vi "Explore States Dialog.vi"(5 "Calling VI Ref":refnum<vi>, 8 "error in (no error)":errorcluster, 9 "StringConstant":refnum<vi>, 11 "JKI SM in":refnum<class "JKI SM.lvclass">) -> (0 "error out":errorcluster)   [LabVIEW 2020]
uses:
  JKI State Machine API/source/JKI SM/JKI SM.lvclass
  <userlib>/_OpenG.lib/error/error.llb/Filter Error Codes (Array)__ogtk.vi
  <vilib>/regexp/Match Regular Expression.xnode
  <userlib>/_OpenG.lib/comparison/comparison.llb/openg_comparison__ogtk.lvlib
  <userlib>/_OpenG.lib/comparison/comparison.llb/I32 Changed__ogtk.vi
  <userlib>/_OpenG.lib/comparison/comparison.llb/Boolean Changed__ogtk.vi
  <userlib>/_OpenG.lib/error/error.llb/openg_error.lvlib
  <userlib>/_OpenG.lib/string/string.llb/openg_string.lvlib
panel:
  in  "Listbox":i32(listbox)
  in  "OK":bool
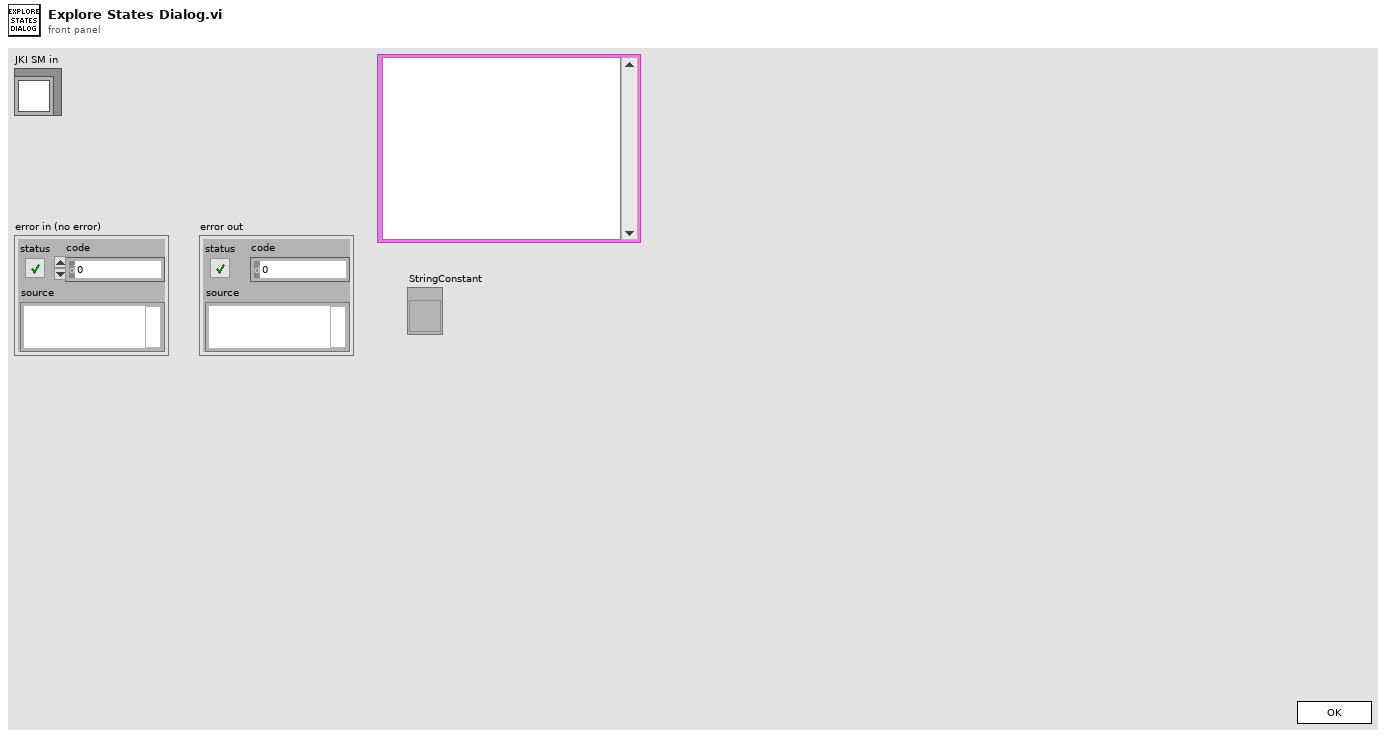
[diagram p1: front panel]
types:
  T1 = enum32{"Invalid", "Standard", "Closed", "Hidden", "Minimized", "Maximized"}
  T2 = enum32{"invalid app kind", "Development System", "Run Time System", "Student Edition", "Embedded LabVIEW", "Evaluation", "Custom"}
  T3 = enum32{"Invalid", "Default", "Floating", "Floating/Auto-Hide", "Modal"}
  T4 = cluster{"Core":cluster{"Current VI Reference":refnum<vi>, "Close Panel on Exit?":bool}, "Your Boolean data":bool, "Originating State":string, "JKI SM out":refnum<class "JKI SM.lvclass">, "States":string[], "StringConstant":refnum<vi>}
  T5 = cluster{"StringConstant":refnum<vi>, "Action":string, "Action":string}
  T6 = typedef "LVPoint32TypeDef.ctl" = cluster{"Horizontal":i32, "Vertical":i32}
  T7 = cluster{"Shift":bool, "Ctrl":bool, "Alt":bool, "Cmd":bool, "Opt":bool}
  T8 = cluster{"StringConstant":refnum<vi>, "Structure":string, "Frame Name":string, "State Call":string}[]
  T9 = cluster{"Current VI Reference":refnum<vi>, "Close Panel on Exit?":bool}
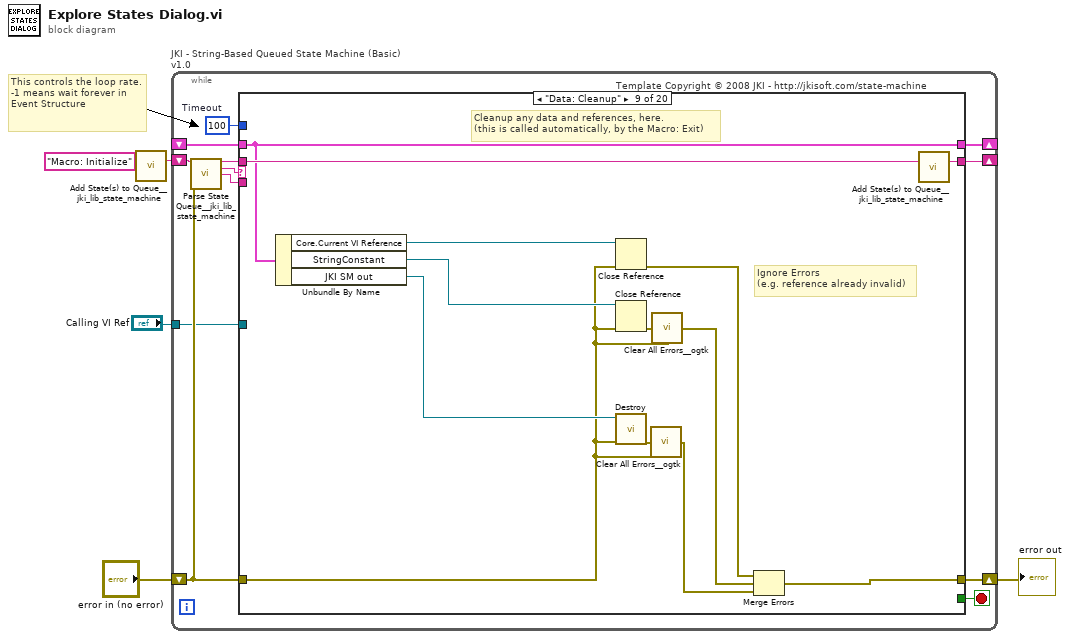
[diagram p0: block diagram]
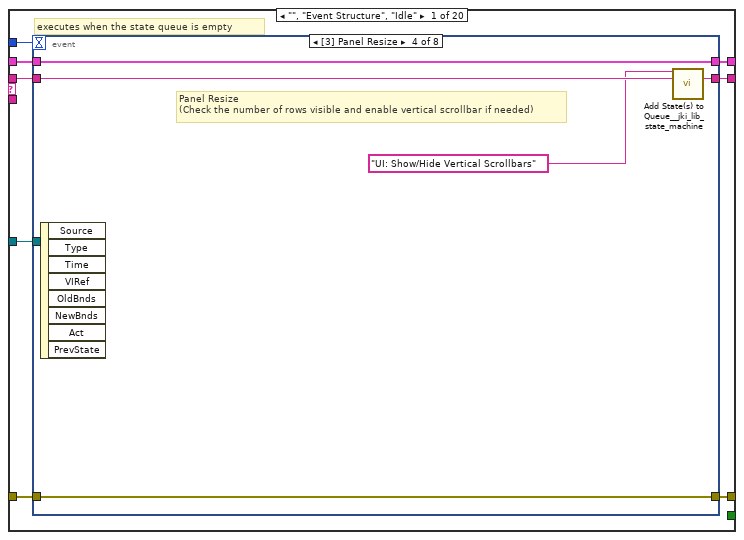
[diagram p2: hidden frame]
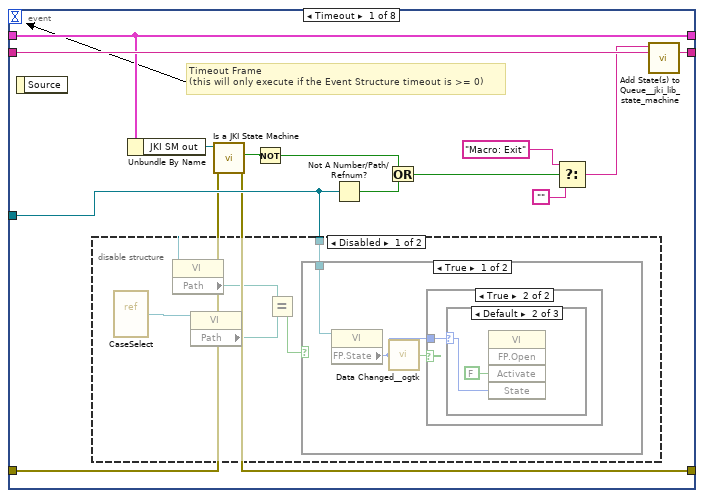
[diagram p3: hidden frame]
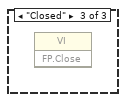
[diagram p6: hidden frame]
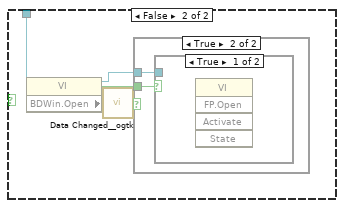
[diagram p7: hidden frame]
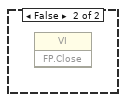
[diagram p9: hidden frame]
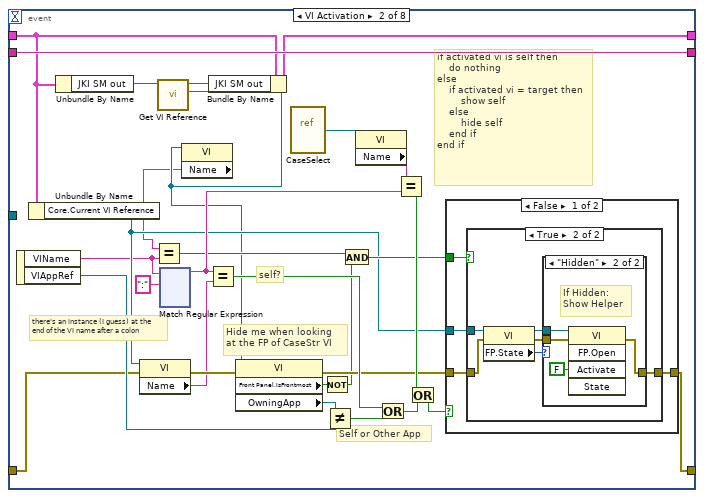
[diagram p11: hidden frame]
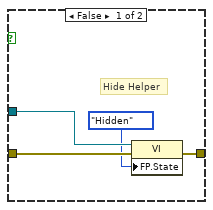
[diagram p12: hidden frame]
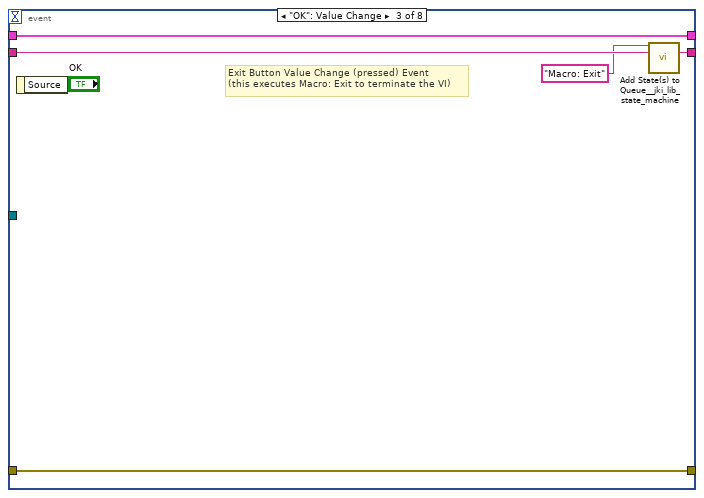
[diagram p15: hidden frame]
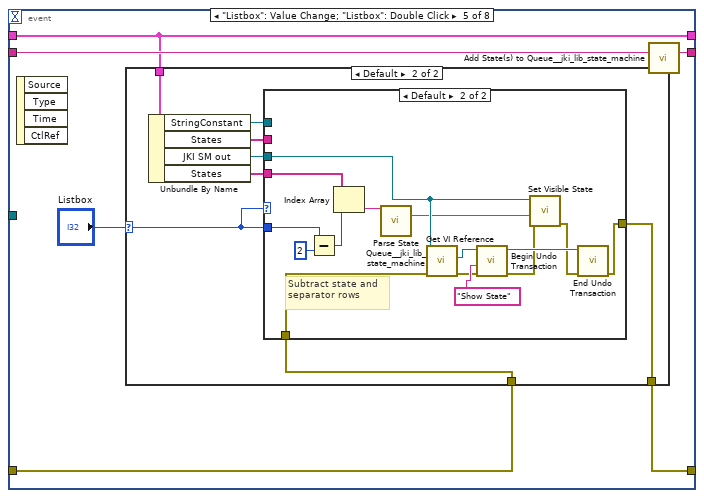
[diagram p16: hidden frame]
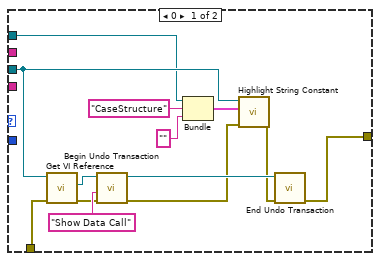
[diagram p18: hidden frame]
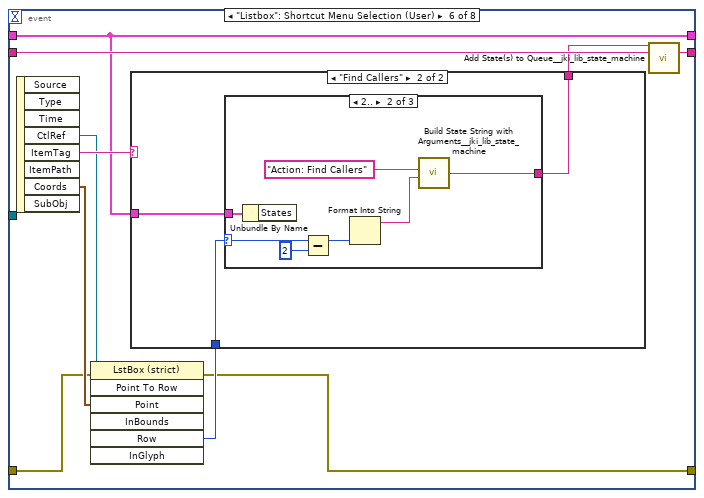
[diagram p19: hidden frame]
diagram:
  # "This controls the loop rate. -1 means wait forever in Event Structure"
  n1 = call <vilib>:"Add State(s) to Queue__jki_lib_state_machine.vi"("State(s) in (\"\")"="Macro: Initialize") -> ("States Out"=w5:string)  [unwired: 14 in]
  n2 = while "JKI - String-Based Queued State Machine (Basic) v1.0" {
    shift-right: [w10] -> _
    shift-left: _ -> [w9]
    shift-right: [w13] -> w3
    shift-left: "error in (no error)" -> [w7]
    shift-right: [w12] -> _
    shift-left: w5 -> [w14]
    tunnel: "Calling VI Ref" -> [w6]
    stop <- w11 stop-if-true
    w8 = 100  # Timeout
    # "Template Copyright © 2008 JKI - http://jkisoft.com/state-machine"
    n3 = call <vilib>:"Parse State Queue__jki_lib_state_machine.vi"("State Queue"=w14, "Error In (no error)"=w7) -> ("Remaining States"=w16:string, "Current State"=w17:string, "Arguments"=w15:string)  [unwired: 11 in]
    n4 = case shown="\"Data: Cleanup\"" w17 {
      selector: w17 -> [_ _ w380 _ _ _ _ _ _ _ _ _ _ _ _ _ _ _ _ _]
      tunnel: w16 -> [w25 w379 w384 w404 w415 w420 w424 w440 w453 w457 w469 w502 w527 w552 w563 w592 w597 w607 w611 w627]
      tunnel: w15 -> [_ _ _ _ _ _ _ _ _ _ _ _ _ w547 w557 _ _ _ _ w625]
      tunnel: w9 -> [w23 w376 w382 w396 w412 w418 w421 _ w450 w454 w461 w499 w521 w550 w559 w589 w595 w604 w608 w622]
      tunnel: [w22 w377 w386 w391 errorcluster {"status"=FALSE, "code"=0, "source"=""} ("error out") w417 w422 w431 w447 w455 w458 w496 w518 w548 w560 w590 w593 w605 w609 w617] -> w13
      tunnel: w7 -> [w21 w377 w385 w392 w410 w417 w422 w426 w442 w455 w459 w492 w519 w549 w561 w590 w593 w605 w609 w614]
      tunnel: [w24 w378 w383 w403 w414 w419 w423 w439 w452 w456 w468 w501 w526 w551 w562 w591 w596 w606 w610 w626] -> w12
      tunnel: [_ _ _ _ _ TRUE _ _ _ _ _ _ _ _ _ _ _ _ _ _] -> w11
      tunnel: [w20 w376 w382 w402 w412 w418 w421 w438 w450 w454 w461 w475 w521 w550 w559 w589 w595 w604 w608 w622] -> w10
      tunnel: w8 -> [w19 _ _ _ _ _ _ _ _ _ _ _ _ _ _ _ _ _ _ _]
      tunnel: w6 -> [w18 _ _ _ _ _ _ _ _ _ _ _ _ _ _ _ _ _ _ w616]
      frame "", "Event Structure", "Idle" {
        # "executes when the state queue is empty"
        n5 = event shown="[3] Panel Resize" {
          selector: _ -> [_ _ _ _ _ _ _ _]
          dyn-events: _ -> [_ _ _ _ _ _ _ _]
          timeout: w19 -> [_ _ _ _ _ _ _ _]
          tunnel: w25 -> [w39 w85 w221 w226 w232 w279 w302 w375]
          tunnel: [w38 w85 w220 w225 w231 w278 w301 w374] -> w24
          tunnel: w23 -> [w33 w59 w218 w223 w230 w270 w300 w372]
          tunnel: [w28 w60 w219 w224 w228 w271 w295 w373] -> w22
          tunnel: w21 -> [w29 w61 w219 w224 w229 w273 w296 w373]
          tunnel: [w33 w58 w218 w223 w230 w270 w300 w372] -> w20
          tunnel: w18 -> [w34 _ _ _ _ _ _ _]
          event Timeout {
            # "Timeout Frame\n(this will only execute if the Event Structure timeout is >= 0)"
            n6 = event-data() -> ()  [unwired: 1 in, 1 out]
            n7 = disable-structure shown="Disabled" {
              disable-tunnel: w34 -> [w40 _]
              frame Disabled {
                n8 = vi-ref "CaseSelect.vi"() -> (w42:refnum<vi>)
                n9 = property class="VI"(reference=w40) -> ("Path"=w41:path)  [unwired: 1 in, 2 out]
                n10 = property class="VI"(reference=w42) -> ("Path"=w44:path)  [unwired: 1 in, 2 out]
                n11 = Equal?(x=w41, y=w44) -> (x = y?=w43:bool)
                n12 = case shown="True" w43 {
                  tunnel: w40 -> [w45 w52]
                  frame True {
                    n13 = property class="VI"(reference=w45) -> ("FP.State"=w46:T1)  [unwired: 1 in, 2 out]
                    n14 = call-poly <userlib>:"Data Changed__ogtk.vi"("I32"=w46) -> ("Changed"=w47:bool)
                    n15 = case shown="True" w47 {
                      tunnel: w46 -> [_ w48]
                      frame False {
                      }
                      frame True {
                        n16 = case shown="Default" w48 {
                          selector: w48 -> [_ w49 _]
                          frame "Invalid" {
                          }
                          frame Default {
                            n17 = invoke class="VI" method="FP.Open"("Activate"=FALSE ("Activate?"), "State"=w49) -> ()  [unwired: 3 in, 5 out]
                          }
                          frame "Closed" {
                            n18 = invoke class="VI" method="FP.Close"() -> ()  [unwired: 3 in, 3 out]
                          }
                        }
                      }
                    }
                  }
                  frame False {
                    n19 = property class="VI"(reference=w52) -> (reference out=w51:refnum<vi>, "BDWin.Open"=w53:bool)  [unwired: 1 in, 1 out]
                    n20 = call-poly <userlib>:"Data Changed__ogtk.vi"("Boolean"=w53) -> ("Changed"=w54:bool)
                    n21 = case shown="True" w54 {
                      tunnel: w53 -> [_ w56]
                      tunnel: w51 -> [_ w55]
                      frame False {
                      }
                      frame True {
                        n22 = case shown="True" w56 {
                          tunnel: w55 -> [_ _]
                          frame True {
                            n23 = invoke class="VI" method="FP.Open"() -> ()  [unwired: 5 in, 5 out]
                          }
                          frame False {
                            n24 = invoke class="VI" method="FP.Close"() -> ()  [unwired: 3 in, 3 out]
                          }
                        }
                      }
                    }
                  }
                }
              }
              frame Enabled {
              }
            }
            n25 = Unbundle By Name(w33) -> ("JKI SM out"=w32:refnum<class "JKI SM.lvclass">)
            n26 = call "Is a JKI State Machine.vi"("error in (no error)"=w29, "JKI SM in"=w32) -> ("error out"=w28:errorcluster, "Is a JKI State Machine"=w31:bool)  [unwired: 7 in, 1 out]
            n27 = Not(x=w31) -> (.not. x?=w30:bool)
            n28 = Not A Number/Path/Refnum?(number/path/refnum=w34) -> (NaN/Path/Refnum?=w27:bool)
            n29 = Or(x=w30, y=w27) -> (x .or. y?=w26:bool)
            n30 = Select(t="Macro: Exit", s=w26, f="") -> (s? t:f=w35:string)
            n31 = call <vilib>:"Add State(s) to Queue__jki_lib_state_machine.vi"("State(s) in Front (\"\")"=w35, "State(s) in (\"\")"=w39) -> ("States Out"=w38:string)  [unwired: 13 in]
          }
          event VI Activation {
            # "Self or Other App"
            # "self?"
            # "Hide me when looking\nat the FP of CaseStr VI"
            # "there's an instance (I guess) at the\nend of the VI name after a colon"
            # "if activated vi is self then\n    do nothing\nelse\n    if activated vi = target then\n        show self\n    else\n        hide self\n    end if\nend if"
            n32 = event-data() -> ("VIName"=w63:string, "VIAppRef"=w62:refnum<vi>)  [unwired: 1 in]
            n33 = Unbundle By Name(w59) -> ("Core.Current VI Reference"=w70:refnum<vi>)
            n34 = Unbundle By Name(w59) -> ("JKI SM out"=w66:refnum<class "JKI SM.lvclass">)
            n35 = property class="VI"(reference=w70, error in=w61) -> (error out=w74:errorcluster, "Name"=w69:string)  [unwired: 1 out]
            n36 = call "Get VI Reference.vi"("JKI SM in"=w66) -> ("VI"=w65:refnum<vi>, "JKI SM out"=w57:refnum<class "JKI SM.lvclass">)  [unwired: 8 in, 1 out]
            n37 = xnode "Match Regular Expression"("input string"=w63, "regular expression"=":") -> ("before match"=w81:string)  [unwired: 3 in, 5 out]
            n38 = property class="VI"(reference=w65) -> ("Name"=w64:string)  [unwired: 1 in, 2 out]
            n39 = Equal?(x=w64, y=w63) -> (x = y?=w67:bool)
            n40 = Equal?(x=w81, y=w69) -> (x = y?=w78:bool)
            n41 = Bundle By Name(cluster=w59, "JKI SM out"=w57) -> (w58:T4)
            n42 = property class="VI"(reference=w65, error in=w74) -> (error out=w73:errorcluster, "Front Panel.IsFrontmost"=w71:bool, "OwningApp"=w76:refnum<vi>)  [unwired: 1 out]
            n43 = vi-ref "CaseSelect.vi"() -> (w79:refnum<vi>)
            n44 = Not(x=w71) -> (.not. x?=w72:bool)
            n45 = Not Equal?(x=w76, y=w62) -> (x != y?=w77:bool)
            n46 = And(x=w67, y=w72) -> (x .and. y?=w75:bool)
            n47 = property class="VI"(reference=w79) -> ("Name"=w80:string)  [unwired: 1 in, 2 out]
            n48 = Or(x=w78, y=w77) -> (x .or. y?=w83:bool)
            n49 = Equal?(x=w80, y=w81) -> (x = y?=w82:bool)
            n50 = Or(x=w82, y=w83) -> (x .or. y?=w84:bool)
            n51 = case shown="False" w84 {
              tunnel: w73 -> [w89 w105]
              tunnel: [w87 w105] -> w60
              tunnel: w70 -> [w88 _]
              tunnel: w75 -> [w86 _]
              frame False {
                n52 = case shown="True" w86 {
                  tunnel: w89 -> [w93 w98]
                  tunnel: w88 -> [w92 w99]
                  tunnel: [w91 w96] -> w87
                  frame False {
                    # "Hide Helper"
                    n53 = property class="VI"(reference=w92, error in=w93, "FP.State"=T1."Hidden" ("Front Panel Window:State")) -> (error out=w91:errorcluster)  [unwired: 1 out]
                  }
                  frame True {
                    n54 = property class="VI"(reference=w99, error in=w98) -> (reference out=w95:refnum<vi>, error out=w94:errorcluster, "FP.State"=w97:T1)
                    n55 = case shown="\"Hidden\"" w97 {
                      tunnel: [w100 w104] -> w96
                      tunnel: w95 -> [_ w103]
                      tunnel: w94 -> [w100 w102]
                      frame Default {
                      }
                      frame "Hidden" {
                        # "If Hidden:\nShow Helper"
                        n56 = invoke class="VI" method="FP.Open"(reference=w103, error in=w102, "Activate"=FALSE ("Activate?")) -> (error out=w104:errorcluster)  [unwired: 2 in, 4 out]
                      }
                    }
                  }
                }
              }
              frame True {
              }
            }
          }
          event "OK": Value Change {
            # "Exit Button Value Change (pressed) Event\n(this executes Macro: Exit to terminate the VI)"
            n57 = event-data() -> ()  [unwired: 1 in, 1 out]
            n58 = call <vilib>:"Add State(s) to Queue__jki_lib_state_machine.vi"("State(s) in Front (\"\")"="Macro: Exit", "State(s) in (\"\")"=w221) -> ("States Out"=w220:string)  [unwired: 13 in]
          }
          event Panel Resize {
            # "Panel Resize\n(Check the number of rows visible and enable vertical scrollbar if needed)"
            n59 = event-data() -> ()  [unwired: 1 in, 8 out]
            n60 = call <vilib>:"Add State(s) to Queue__jki_lib_state_machine.vi"("State(s) in Front (\"\")"="UI: Show/Hide Vertical Scrollbars" ("State(s) in Front (\"\")"), "State(s) in (\"\")"=w226) -> ("States Out"=w225:string)  [unwired: 13 in]
          }
          event "Listbox": Value Change; "Listbox": Double Click {
            n61 = event-data() -> ()  [unwired: 1 in, 4 out]
            n62 = case shown="Default" "Listbox" {
              selector: "Listbox" -> [_ w235]
              tunnel: w230 -> [_ w241]
              tunnel: w229 -> [w233 w238]
              tunnel: [w233 w237] -> w228
              frame -1 {
              }
              frame Default {
                n63 = Unbundle By Name(w241) -> ("StringConstant"=w234:refnum<vi>, "States"=w236:string[], "JKI SM out"=w239:refnum<class "JKI SM.lvclass">, "States"=w240:string[])
                n64 = case shown="Default" w235 {
                  tunnel: w240 -> [_ w269]
                  tunnel: w239 -> [w253 w262]
                  tunnel: w238 -> [w254 w258]
                  tunnel: w235 -> [_ w267]
                  tunnel: [w252 w259] -> w237
                  tunnel: w236 -> [_ _]
                  tunnel: w234 -> [w251 _]
                  frame 0 {
                    n65 = call "Get VI Reference.vi"("error in (no error)"=w254, "JKI SM in"=w253) -> ("error out"=w249:errorcluster, "VI"=w248:refnum<vi>)  [unwired: 7 in, 1 out]
                    n66 = call "Begin Undo Transaction.vi"("error in (no error)"=w249, "Action"="Show Data Call", "VI in"=w248) -> ("error out"=w245:errorcluster, "VI out"=w247:refnum<vi>)  [unwired: 7 in]
                    n67 = Bundle("StringConstant"=w251, "Action"="CaseStructure", "Action"="") -> (w244:T5)  [unwired: 1 in]
                    n68 = call "Highlight String Constant.vi"("error in (no error)"=w245, "Cluster"=w244, "JKI SM in"=w253) -> ("error out"=w246:errorcluster)  [unwired: 7 in, 1 out]
                    n69 = call "End Undo Transaction.vi"("error in (no error)"=w246, "VI in"=w247) -> ("error out"=w252:errorcluster)  [unwired: 8 in, 1 out]
                  }
                  frame Default {
                    # "Subtract state and separator rows"
                    n70 = Subtract(x=w267, y=2) -> (x-y=w266:i32)
                    n71 = Index Array(array=w269, index=w266) -> (element=w256:string)
                    n72 = call <vilib>:"Parse State Queue__jki_lib_state_machine.vi"("State Queue"=w256) -> ("Current State"=w255:string)  [unwired: 12 in, 2 out]
                    n73 = call "Get VI Reference.vi"("error in (no error)"=w258, "JKI SM in"=w262) -> ("error out"=w264:errorcluster, "VI"=w263:refnum<vi>)  [unwired: 7 in, 1 out]
                    n74 = call "Begin Undo Transaction.vi"("error in (no error)"=w264, "Action"="Show State", "VI in"=w263) -> ("error out"=w257:errorcluster, "VI out"=w261:refnum<vi>)  [unwired: 7 in]
                    n75 = call "Set Visible State.vi"("error in (no error)"=w257, "State Name"=w255, "JKI SM in"=w262) -> ("error out"=w260:errorcluster)  [unwired: 7 in, 1 out]
                    n76 = call "End Undo Transaction.vi"("error in (no error)"=w260, "VI in"=w261) -> ("error out"=w259:errorcluster)  [unwired: 8 in, 1 out]
                  }
                }
              }
            }
            n77 = call <vilib>:"Add State(s) to Queue__jki_lib_state_machine.vi"("State(s) in (\"\")"=w232) -> ("States Out"=w231:string)  [unwired: 14 in]
          }
          event "Listbox": Shortcut Menu Selection (User) {
            n78 = event-data() -> ("CtlRef"=w276:refnum<vi>, "ItemTag"=w277:string, "Coords"=w275:T6)  [unwired: 1 in, 5 out]
            n79 = invoke class="LstBox (strict)" method="Point To Row"(reference=w276, error in=w273, "Point"=w275) -> (error out=w271:errorcluster, "Row"=w274:i32)  [unwired: 4 in, 5 out]
            n80 = case shown="\"Find Callers\"" w277 {
              tunnel: w274 -> [_ w282]
              tunnel: [_ w281] -> w272
              tunnel: w270 -> [_ w280]
              frame Default {
              }
              frame "Find Callers" {
                n81 = case shown="2.." w282 {
                  selector: w282 -> [_ w286 _]
                  tunnel: [_ w287 w290] -> w281
                  tunnel: w280 -> [_ w283 _]
                  frame -1, Default {
                  }
                  frame 2.. {
                    n82 = Unbundle By Name(w283) -> ()  [unwired: 1 out]
                    n83 = Subtract(x=w286, y=2) -> (x-y=w285:i32)
                    n84 = Format Into String(w285) -> (resulting string=w288:string)  [unwired: 3 in, 1 out]
                    n85 = call <vilib>:"Build State String with Arguments__jki_lib_state_machine.vi"("Arguments (\"\")"=w288, "State"="Action: Find Callers") -> ("State with Arguments"=w287:string)  [unwired: 4 in]
                  }
                  frame 0 {
                    n86 = disable-structure shown="Disabled" {
                      disable-tunnel: [w291 _] -> w290
                      frame Disabled {
                        n87 = call <vilib>:"Build State String with Arguments__jki_lib_state_machine.vi"("State"="Action: Delete State") -> ("State with Arguments"=w291:string)  [unwired: 5 in]
                      }
                      frame Enabled {
                      }
                    }
                  }
                }
              }
            }
            n88 = call <vilib>:"Add State(s) to Queue__jki_lib_state_machine.vi"("State(s) in Front (\"\")"=w272, "State(s) in (\"\")"=w279) -> ("States Out"=w278:string)  [unwired: 13 in]
          }
          event Key Down? {
            n89 = event-data() -> ("Char"=w299:i16, "ScanCode"=w294:i16, "PlatMods"=w298:T7)  [unwired: 1 in, 7 out]
            n90 = case shown="Default" w294 {
              tunnel: w300 -> [_ w320]
              tunnel: w299 -> [_ w318]
              tunnel: w298 -> [_ w315]
              tunnel: [_ w313] -> w297
              tunnel: w296 -> [w304 w311]
              tunnel: [w304 w310] -> w295
              tunnel: [w303 _] -> w293
              frame 83 {
                n91 = local read "Listbox"() -> (w305:i32)
                n92 = case shown="Default" w305 {
                  selector: w305 -> [_ w306]
                  tunnel: [_ w307] -> w303
                  frame -1 {
                  }
                  frame Default {
                    n93 = Format Into String(w306) -> (resulting string=w308:string)  [unwired: 3 in, 1 out]
                    n94 = call <vilib>:"Build State String with Arguments__jki_lib_state_machine.vi"("Arguments (\"\")"=w308, "State"="Action: Delete State Call") -> ("State with Arguments"=w307:string)  [unwired: 4 in]
                  }
                }
              }
              frame Default {
                n95 = Unbundle By Name(w320) -> ("JKI SM out"=w312:refnum<class "JKI SM.lvclass">, "States"=w319:string[])
                n96 = Build Array(w318) -> (w317:i16[])
                n97 = Unbundle By Name(w315) -> ("Ctrl"=w314:bool)
                n98 = Byte Array To String(unsigned byte array=w317) -> (string=w316:string)
                n99 = case shown="True" w314 {
                  tunnel: w319 -> [_ w329]
                  tunnel: w316 -> [_ w328]
                  tunnel: w315 -> [_ w327]
                  tunnel: [_ w326] -> w313
                  tunnel: w312 -> [_ w324]
                  tunnel: [w321 w323] -> w310
                  tunnel: w311 -> [w321 w322]
                  frame False {
                  }
                  frame True {
                    n100 = To Upper Case(1:w328) -> (0:w325:string)
                    n101 = case shown="\"F\"" w325 {
                      tunnel: w329 -> [_ w344 w353 _]
                      tunnel: w327 -> [_ w339 _ w362]
                      tunnel: [_ TRUE TRUE TRUE] -> w326
                      tunnel: w324 -> [_ _ w347 w359]
                      tunnel: [w330 w337 w345 w356] -> w323
                      tunnel: w322 -> [w330 w337 w346 w360]
                      frame Default {
                      }
                      frame "G" {
                        w332 = 2 ("y")
                        n102 = local read "Listbox"() -> (w334:i32)
                        n103 = Unbundle By Name(w339) -> ("Shift"=w340:bool)
                        n104 = Array Size(array=w344) -> (size(s)=w331:i32)
                        n105 = Subtract(x=w334, y=w332) -> (x-y=w333:i32)
                        n106 = Decrement(x=w333) -> (x-1=w342:i32)
                        n107 = Increment(x=w333) -> (x+1=w343:i32)
                        n108 = Select(t=w342, s=w340, f=w343) -> (s? t:f=w341:i32)
                        n109 = Quotient & Remainder(x=w341, y=w331) -> (x-y*floor(x/y)=w336:i32)  [unwired: 1 out]
                        n110 = Add(x=w336, y=w332) -> (x+y=w335:i32)
                        n111 = property on="Listbox" class="LstBox (strict)"("Val(Sgnl)"=w335) -> ()  [unwired: 2 in, 2 out]
                      }
                      frame "F" {
                        n112 = local read "Listbox"() -> (w354:i32)
                        n113 = Index Array(array=w353, index=w354) -> (element=w352:string)
                        n114 = control-ref of="This VI"() -> (w348:refnum<vi>)
                        n115 = call "Find All Callers of State.vi"("error in (no error)"=w346, "State Name"=w352, "JKI SM in"=w347) -> ("error out"=w349:errorcluster, "Callers"=w350:T8, "JKI SM out"=w351:refnum<class "JKI SM.lvclass">)  [unwired: 6 in]
                        n116 = call "Open Search Results Dialog.vi"("VI Refnum"=w348, "error in (no error)"=w349, "Callers"=w350, "State"=w352, "JKI SM in"=w351) -> ("error out"=w345:errorcluster)  [unwired: 6 in]
                      }
                      frame "Z" {
                        # "Override Ctrl+Z and Ctrl+Shift+Z\n(Handle them here and target the user's VI)"
                        n117 = call "Get VI Reference.vi"("error in (no error)"=w360, "JKI SM in"=w359) -> ("error out"=w357:errorcluster, "VI"=w358:refnum<vi>)  [unwired: 7 in, 1 out]
                        n118 = Unbundle By Name(w362) -> ("Shift"=w361:bool)
                        n119 = case shown="False" w361 {
                          tunnel: w358 -> [w366 w369]
                          tunnel: w357 -> [w364 w368]
                          tunnel: [w365 w367] -> w356
                          frame False {
                            n120 = invoke class="VI" method="Transaction.Undo"(reference=w366, error in=w364) -> (error out=w365:errorcluster)  [unwired: 1 in, 2 out]
                          }
                          frame True {
                            n121 = invoke class="VI" method="Transaction.Redo"(reference=w369, error in=w368) -> (error out=w367:errorcluster)  [unwired: 1 in, 2 out]
                          }
                        }
                      }
                    }
                  }
                }
              }
            }
            n122 = event-data("Discard?"=w297) -> ()  [unwired: 1 in, 1 out]
            n123 = call <vilib>:"Add State(s) to Queue__jki_lib_state_machine.vi"("State(s) in Front (\"\")"=w293, "State(s) in (\"\")"=w302) -> ("States Out"=w301:string)  [unwired: 13 in]
          }
          event Panel Close? {
            # "Discard the event because we'll close the front panel ourselves in Macro: Exit"
            # "Close Panel button (pressed) Event\n(this executes Macro: Exit to terminate the VI)"
            n124 = event-data() -> ()  [unwired: 1 in, 1 out]
            n125 = event-data("Discard?"=TRUE) -> ()  [unwired: 1 in, 1 out]
            n126 = call <vilib>:"Add State(s) to Queue__jki_lib_state_machine.vi"("State(s) in Front (\"\")"="Macro: Exit", "State(s) in (\"\")"=w375) -> ("States Out"=w374:string)  [unwired: 13 in]
          }
        }
      }
      frame "---------- Core ----------" {
        # "Do not put any code in this frame.\n(it is a separator no-op)"
        n127 = call <vilib>:"Add State(s) to Queue__jki_lib_state_machine.vi"("State(s) in (\"\")"=w379) -> ("States Out"=w378:string)  [unwired: 14 in]
      }
      frame Default {
        w389 = 42 items=["No error", "Argument error", "Memory is full", "Out of zone", "End of file", "File already open", "Generic file I/O error", "File not found", "File permission error", "Disk is full", "Duplicate path", "Too many files open", "System feature not enabled", "Resource file not found", "Cannot add resource", "Resource not found", "Image not found", "Image memory error", "Pen does not exist", "Config type invalid", "Config token not found", "Config parse error", "Config memory error", "Bad external code format", "Bad external code offset", "External code not present", "Null window", "Destroy window error", "Null menu", "Print aborted", "Bad print record", "Print driver error", "Windows error during printing", "Memory error during printing", "Print dialog error", "Generic print error", "Invalid device refnum", "Device not found", "Device parameter error", "Device unit error", "Cannot open device", "Device call aborted", "Generic error", "Cancelled by user", "Object ID too low", "Object ID too high", "Object not in heap", "Unknown heap", "Unknown object (invalid DefProc)", "Unknown object (DefProc not in table)", "Message out of range", "Invalid (null) method", "Unknown message", "Manager call not supported", "Bad address", "Network operation in progress", "Network operation timed out", "Connection is busy", "Network attribute not supported", "Network error", "Address in use", "System out of memory", "Connection aborted", "Connection refused", "Not connected", "Already connected", "Connection closed", "Initialization error (interapplication manager)", "Bad occurrence", "Wait on unbound occurrence handler", "Occurrence queue overflow", "Datalog type conflict", "Unused", "Unrecognized type (interapplication manager)", "Memory corrupt", "Failed to make temporary DLL", "Old CIN version", "Drag socket not found", "Failed to load drop-object", "Failed to register OLE object", "Failed to release OLE object", "Format specifier type mismatch", "Unknown format specifier", "Too few format specifiers", "Too many format specifiers", "Scan failed", "Newer CIN version", "Error converting to variant", "Runtime menu error", "Password tampered", "Variant attribute not found", "Incompatible variant data type", "Event data is not available", "Event Store is not present", "Occurrence is not found", "Event Queue is not created", "Event info is not available", "Refnum passed is NULL", "Error retrieving Class GUID", "Error retrieving CoClass GUID", "Error retrieving TypeLib GUID.", "Bad built application magic bytes.", "Specific driver is different from the specific driver associated with the Logical Name.", "There is no session opened to the class driver.", "Max Error", "MAX - Error with config objects", "MAX - Error loading configuration", "MAX - Group not supported"]
        # "Current State"
        # "Do not delete, rename, or modify this frame.\n(this is used to capture unhandled states and typos)"
        # "Handle mistyped state name (developer tool)"
        n128 = Format Into String(format string="Software Exception: Unhandled State \"%s\"." ("message"), error in=w385, w380) -> (resulting string=w388:string, error out=w387:errorcluster)  [unwired: 1 in]
        n129 = call <vilib>:"Error Cluster From Error Code.vi"("show call chain? (False)"=TRUE, "error in (no error)"=w387, "error message (\"\")"=w388, "error code (0)"=w389) -> ("error out"=w386:errorcluster)  [unwired: 5 in]
        n130 = call <vilib>:"Add State(s) to Queue__jki_lib_state_machine.vi"("State(s) in (\"\")"=w384) -> ("States Out"=w383:string)  [unwired: 14 in]
      }
      frame "Initialize Core Data" {
        # "Do not delete, rename, or modify this frame.\n(this is used to determine panel behavior on exit)"
        # "originally closed?"
        # "exe?"
        # "If panel starts closed or is an EXE, then close it when we exit"
        n131 = property class="VI"() -> ("Clone Name"=w394:string)  [unwired: 2 in, 2 out]
        n132 = Open VI Reference(vi path=w394, error in (no error)=w392) -> (vi reference=w393:refnum<vi>, error out=w391:errorcluster)  [unwired: 4 in]
        n133 = property class="VI"() -> ("Front Panel.Open"=w401:bool)  [unwired: 2 in, 2 out]
        n134 = property class="App"() -> ("App.Kind"=w400:T2)  [unwired: 2 in, 2 out]
        n135 = Not(x=w401) -> (.not. x?=w398:bool)
        n136 = Equal?(x=w400, y=T2."Run Time System" ("Application:Kind")) -> (x = y?=w397:bool)
        n137 = Or(x=w398, y=w397) -> (x .or. y?=w395:bool)
        n138 = Bundle By Name(cluster=w396, "Core.Current VI Reference"=w393, "Core.Close Panel on Exit?"=w395) -> (w402:T4)
        n139 = call <vilib>:"Add State(s) to Queue__jki_lib_state_machine.vi"("State(s) in (\"\")"=w404) -> ("States Out"=w403:string)  [unwired: 14 in]
      }
      frame "Error Handler" {
        w411 = i32[] [1026]  # JKI SM VI Invalid Ref
        # "Unhandled Error -- Display it"
        # "Handle any errors here.\nYou can also output any states to clean-up after errors occur"
        # "Clear error"
        n140 = call-poly <userlib>:"Filter Error Codes__ogtk.vi"("Error In"=w410, "Error Codes to Filter"=w411) -> ("Error Out"=w409:errorcluster, "Error Filtered?"=w408:bool)  [unwired: 7 in, 1 out]
        n141 = call <vilib>:"General Error Handler.vi"("error in (no error)"=w409) -> ()  [unwired: 10 in, 5 out]
        n142 = Select(t="Macro: Exit", s=w408, f="") -> (s? t:f=w405:string)
        n143 = call <vilib>:"Add State(s) to Queue__jki_lib_state_machine.vi"("State(s) in Front (\"\")"=w405, "State(s) in (\"\")"=w415) -> ("States Out"=w414:string)  [unwired: 13 in]
      }
      frame "Exit" {
        # "Do not put any code in this frame.\n(No errors that occur here will be handled.)"
        n144 = call <vilib>:"Add State(s) to Queue__jki_lib_state_machine.vi"("State(s) in (\"\")"=w420) -> ("States Out"=w419:string)  [unwired: 14 in]
      }
      frame "---------- Data ----------" {
        # "Do not put any code in this frame.\n(It is a separator no-op. You can make a copy of this frame to create a new Data frame)"
        n145 = call <vilib>:"Add State(s) to Queue__jki_lib_state_machine.vi"("State(s) in (\"\")"=w424) -> ("States Out"=w423:string)  [unwired: 14 in]
      }
      frame "Data: Initialize" {
        w434 = string[] []  # States
        w435 = T9 {"Current VI Reference"=refnum, "Close Panel on Exit?"=FALSE}  # Core
        w437 = TRUE  # Your Boolean data
        w436 = ""  # Originating State
        # "do not delete - used by framework"
        # "Expand Bundle to add new data elements to shift register data."
        # "Add new data here."
        # "Data names and types of shift register data are defined by this bundle."
        # "Initialize the shift-register data, here.\n(data names are defined by what you wire into the bundle function)"
        n146 = call "Create (From State String Constant).vi"("error in (no error)"=w426, "State String Constant"="StringConstant") -> ("error out"=w425:errorcluster, "JKI SM out"=w427:refnum<class "JKI SM.lvclass">)  [unwired: 6 in, 2 out]
        n147 = property class="StrCnst"(reference="StringConstant", error in=w425) -> (error out=w432:errorcluster, "Text.Text"=w430:string)  [unwired: 1 out]
        n148 = call <userlib>:"Multi-line String to Array__ogtk.vi"("string"=w430) -> ("lines"=w429:string[])
        n149 = Variant To Data(error in=w432, type=w434, Variant=w429) -> (data=w433:string[], error out=w431:errorcluster)
        n150 = Bundle("Core"=w435, "Your Boolean data"=w437, "Originating State"=w436, "JKI SM out"=w427, "States"=w433, "StringConstant"="StringConstant") -> (w438:T4)  [unwired: 1 in]
        n151 = call <vilib>:"Add State(s) to Queue__jki_lib_state_machine.vi"("State(s) in (\"\")"=w440) -> ("States Out"=w439:string)  [unwired: 14 in]
      }
      frame "Data: Cleanup" {
        # "Ignore Errors\n(e.g. reference already invalid)"
        # "Cleanup any data and references, here.\n(this is called automatically, by the Macro: Exit)"
        n152 = Unbundle By Name(w450) -> ("Core.Current VI Reference"=w451:refnum<vi>, "StringConstant"=w449:refnum<vi>, "JKI SM out"=w443:refnum<class "JKI SM.lvclass">)
        n153 = Close Reference(reference=w451, error in (no error)=w442) -> (error out=w448:errorcluster)
        n154 = Close Reference(reference=w449, error in (no error)=w442) -> (error out=w446:errorcluster)
        n155 = call "Destroy.vi"("error in (no error)"=w442, "JKI SM in"=w443) -> ("error out"=w444:errorcluster)  [unwired: 9 in]
        n156 = call <userlib>:"Clear All Errors__ogtk.vi"("Upsteam Error (optional)"=w442, "Error In"=w444) -> ("Error Out"=w441:errorcluster)  [unwired: 2 in]
        n157 = call <userlib>:"Clear All Errors__ogtk.vi"("Upsteam Error (optional)"=w442, "Error In"=w446) -> ("Error Out"=w445:errorcluster)  [unwired: 2 in]
        n158 = Merge Errors(w448, w445, w441) -> (w447:errorcluster)
        n159 = call <vilib>:"Add State(s) to Queue__jki_lib_state_machine.vi"("State(s) in (\"\")"=w453) -> ("States Out"=w452:string)  [unwired: 14 in]
      }
      frame "---------- UI ----------" {
        # "Do not put any code in this frame.\n(It is a separator no-op. You can make a copy of this frame to create a new UI frame)"
        n160 = call <vilib>:"Add State(s) to Queue__jki_lib_state_machine.vi"("State(s) in (\"\")"=w457) -> ("States Out"=w456:string)  [unwired: 14 in]
      }
      frame "UI: Show/Hide Vertical Scrollbars" {
        # "Add +1 for the Parent Frame and another +1 for the horizontal divider"
        n161 = Unbundle By Name(w461) -> ("States"=w464:string[])
        n162 = Array Size(array=w464) -> (size(s)=w467:i32)
        n163 = property on="Listbox" class="LstBox (strict)"(error in=w459) -> (error out=w460:errorcluster, "Number of Rows"=w466:u32)  [unwired: 1 in, 1 out]
        n164 = Increment(x=w467) -> (x+1=w463:i32)
        n165 = Increment(x=w463) -> (x+1=w462:i32)
        n166 = Greater Or Equal?(x=w462, y=w466) -> (x >= y?=w465:bool)
        n167 = property on="Listbox" class="LstBox (strict)"(error in=w460, "Scrollbar Visible"=w465) -> (error out=w458:errorcluster)  [unwired: 1 in, 1 out]
        n168 = call <vilib>:"Add State(s) to Queue__jki_lib_state_machine.vi"("State(s) in (\"\")"=w469) -> ("States Out"=w468:string)  [unwired: 14 in]
      }
      frame "UI: Initialize" {
        # "Initialize the User Interface, here.\n(this is called automatically, by the Macro: Init)"
        n169 = Unbundle By Name(w499) -> ("Core.Current VI Reference"=w500:refnum<vi>, "States"=w471:string[], "JKI SM out"=w497:refnum<class "JKI SM.lvclass">, "StringConstant"=w498:refnum<vi>)
        n170 = property class="StrCnst"(reference=w498, error in=w492) -> (error out=w491:errorcluster, "Label.Text"=w488:string)  [unwired: 1 out]
        n171 = Empty String/Path?(string/path=w488) -> (empty?=w495:bool)
        n172 = call "Get State String Info.vi"("error in (no error)"=w491, "GObj Refnum in"=w498, "JKI SM in"=w497) -> ("error out"=w496:errorcluster, "Frame Name"=w490:string, "Structure"=w482:string)  [unwired: 5 in, 1 out]
        n173 = Not(x=w495) -> (.not. x?=w493:bool)
        n174 = Not Equal?(x=w490, y=w488) -> (x != y?=w494:bool)
        n175 = Equal?(x="EventStructure", y=w482) -> (x = y?=w483:bool)
        n176 = And(x=w494, y=w493) -> (x .and. y?=w489:bool)
        n177 = Build Array(w488) -> (w487:string[])
        n178 = Build Array(w482) -> (w481:string[])
        n179 = Select(t=w487, s=w489, f=string[] []) -> (s? t:f=w486:string[])
        n180 = Select(t=w481, s=w483, f=string[] []) -> (s? t:f=w479:string[])
        n181 = Build Array (concatenate)(w479, w490, w486) -> (w478:string[])
        n182 = call <userlib>:"1D Array to String__ogtk.vi"("delimiter (Tab)"=": ", "Array of Strings"=w478) -> ("delimited string"=w474:string)  [unwired: 9 in]
        n183 = Format Into String(format string="Back to %s", w474) -> (resulting string=w472:string)  [unwired: 2 in, 1 out]
        n184 = disable-structure shown="Enabled" {
          disable-tunnel: w471 -> [w504 w513]
          disable-tunnel: w472 -> [w503 _]
          frame Enabled {
            n185 = Build Array (concatenate)(w503, "" ("format string"), w504) -> (w510:string[])
            n186 = property on="Listbox" class="LstBox (strict)"("Item Names"=w510, "Value"=-1 ("Listbox")) -> (error out=w509:errorcluster, "Item Symbols"=w508:i32[])  [unwired: 2 in, 1 out]
            n187 = Replace Array Subset(array=w508, new element=-1 ("new element/subarray"), index=1) -> (w507:i32[])
            n188 = property on="Listbox" class="LstBox (strict)"(error in=w509, "Item Symbols"=w507) -> ()  [unwired: 1 in, 2 out]
          }
          frame Disabled {
            n189 = Build Array (concatenate)(w513) -> (w516:string[])
            n190 = property on="Listbox" class="LstBox (strict)"("Item Names"=w516, "Value"=-1 ("Listbox")) -> (error out=w515:errorcluster, "Item Symbols"=w514:i32[])  [unwired: 2 in, 1 out]
            n191 = property on="Listbox" class="LstBox (strict)"(error in=w515, "Item Symbols"=w514) -> ()  [unwired: 1 in, 2 out]
          }
        }
        n192 = property class="VI"(reference=w500, "Front Panel.Title"="String Constant" ("format string")) -> ()  [unwired: 1 in, 2 out]
        n193 = Bundle By Name(cluster=w499, "Originating State"=w474) -> (w475:T4)
        n194 = call <vilib>:"Add State(s) to Queue__jki_lib_state_machine.vi"("State(s) in Front (\"\")"="UI: Show/Hide Vertical Scrollbars" ("State(s) in Front (\"\")"), "State(s) in (\"\")"=w502) -> ("States Out"=w501:string)  [unwired: 13 in]
      }
      frame "UI: Pre-Test for 0 or 1 Items" {
        n195 = Unbundle By Name(w521) -> ("JKI SM out"=w522:refnum<class "JKI SM.lvclass">, "JKI SM out"=w524:refnum<class "JKI SM.lvclass">, "States"=w523:string[])
        n196 = Array Size(array=w523) -> (size(s)=w525:i32)
        n197 = case shown="1" w525 {
          tunnel: w524 -> [_ w531 _]
          tunnel: [_ "Macro: Exit" w540] -> w520
          tunnel: w523 -> [_ _ w539]
          tunnel: w522 -> [_ _ w538]
          tunnel: w519 -> [w528 w529 w537]
          tunnel: [w528 w529 w536] -> w518
          frame Default {
          }
          frame 0 {
            n198 = disable-structure shown="Disabled" {
              disable-tunnel: w531 -> [w534 _]
              frame Disabled {
                n199 = Format Into String(format string="State %s has no callers.", w534) -> (resulting string=w532:string)  [unwired: 2 in, 1 out]
                n200 = One Button Dialog(message=w532) -> ()  [unwired: 1 in, 1 out]
              }
              frame Enabled {
              }
            }
          }
          frame 1 {
            n201 = Index Array(array=w539) -> (element=w535:string)  [unwired: 1 in]
            n202 = disable-structure shown="Disabled" {
              disable-tunnel: ["Macro: Exit" _] -> w540
              disable-tunnel: w538 -> [w544 _]
              disable-tunnel: w537 -> [w543 w546]
              disable-tunnel: [w542 w546] -> w536
              disable-tunnel: w535 -> [w541 _]
              frame Disabled {
                # "Just goto state"
                n203 = call "Set Visible State.vi"("error in (no error)"=w543, "State Name"=w541, "JKI SM in"=w544) -> ("error out"=w542:errorcluster)  [unwired: 7 in, 1 out]
              }
              frame Enabled {
                # "Open Dialog - Even if only 1 state"
              }
            }
          }
        }
        n204 = call <vilib>:"Add State(s) to Queue__jki_lib_state_machine.vi"("State(s) in Front (\"\")"=w520, "State(s) in (\"\")"=w527) -> ("States Out"=w526:string)  [unwired: 13 in]
      }
      frame "UI: Cursor Set" {
        # "Argument"
        # "Set and Unset Cursor Busy.\n(Usage: \"UI: Cursor Set >> Busy|Idle\")"
        n205 = case shown="\"Idle\", Default" w547 {
          tunnel: w549 -> [w554 w556]
          tunnel: [w553 w555] -> w548
          frame "Idle", Default {
            n206 = call <vilib>:"Unset Busy.vi"("error in (no error)"=w554) -> ("error out"=w553:errorcluster)  [unwired: 10 in]
          }
          frame "Busy" {
            n207 = call <vilib>:"Set Busy.vi"("error in (no error)"=w556) -> ("error out"=w555:errorcluster)  [unwired: 9 in, 1 out]
          }
        }
        n208 = call <vilib>:"Add State(s) to Queue__jki_lib_state_machine.vi"("State(s) in (\"\")"=w552) -> ("States Out"=w551:string)  [unwired: 14 in]
      }
      frame "UI: Front Panel State" {
        # "Argument"
        # "Set Front Panel Open or Closed\n(Usage: \"UI: Front Panel State >> Open|Close\")"
        n209 = Unbundle By Name(w559) -> ("Core.Current VI Reference"=w558:refnum<vi>)
        n210 = case shown="\"Open\", Default" w557 {
          tunnel: w561 -> [w567 w583]
          tunnel: [w569 w584] -> w560
          tunnel: w558 -> [w568 w581]
          frame "Open", Default {
            n211 = property class="VI"(reference=w568, error in=w567) -> (reference out=w565:refnum<vi>, error out=w566:errorcluster, "Front Panel.Open"=w564:bool)
            n212 = case shown="False" w564 {
              tunnel: [w572 w578] -> w569
              tunnel: w566 -> [w575 w578]
              tunnel: w565 -> [w574 _]
              frame False {
                # "Setting Floatin here, instead of VI Properties allows the VI to accept keyboard input immediately after openning. (setting it in VI Properties was causing a bug where it wouldn't receive keyboard input until clicking on the VI)"
                n213 = invoke class="VI" method="FP.Open"(reference=w574, error in=w575, "Activate"=TRUE, "State"=T1."Standard") -> (reference out=w571:refnum<vi>, error out=w573:errorcluster)  [unwired: 1 in, 3 out]
                n214 = property class="VI"(reference=w571, error in=w573, "FP.Behavior"=T3."Floating" ("Front Panel Window:Behavior")) -> (error out=w572:errorcluster)  [unwired: 1 out]
              }
              frame True {
              }
            }
          }
          frame "Close" {
            n215 = property class="VI"(reference=w581, error in=w583) -> (reference out=w580:refnum<vi>, error out=w582:errorcluster, "Front Panel.Open"=w579:bool)
            n216 = case shown="True" w579 {
              tunnel: [w585 w588] -> w584
              tunnel: w582 -> [w585 w587]
              tunnel: w580 -> [_ w586]
              frame False {
              }
              frame True {
                n217 = invoke class="VI" method="FP.Close"(reference=w586, error in=w587) -> (error out=w588:errorcluster)  [unwired: 1 in, 2 out]
              }
            }
          }
        }
        n218 = call <vilib>:"Add State(s) to Queue__jki_lib_state_machine.vi"("State(s) in (\"\")"=w563) -> ("States Out"=w562:string)  [unwired: 14 in]
      }
      frame "---------- Macro ----------" {
        # "Do not put any code in this frame.\n(It is a separator no-op. You can make a copy of this frame to create a new Macro frame)"
        n219 = call <vilib>:"Add State(s) to Queue__jki_lib_state_machine.vi"("State(s) in (\"\")"=w592) -> ("States Out"=w591:string)  [unwired: 14 in]
      }
      frame "Macro: Initialize" {
        w594 = "Data: Initialize\nInitialize Core Data\nUI: Pre-Test for 0 or 1 Items\nUI: Initialize\nUI: Front Panel State >> Open"  # Data: Initialize Initialize Core Data UI: Pre-Test for 0 or 1 Items UI: Initialize UI: Front Panel State >> Open
        # "Initialization Macro\n(This is called once, when the VI starts)"
        n220 = call <vilib>:"Add State(s) to Queue__jki_lib_state_machine.vi"("State(s) in Front (\"\")"=w594, "State(s) in (\"\")"=w597) -> ("States Out"=w596:string)  [unwired: 13 in]
      }
      frame "Macro: Exit" {
        # "Exit Macro\n(This is called once, when the VI exits)"
        n221 = Unbundle By Name(w604) -> ("Core.Close Panel on Exit?"=w603:bool)
        n222 = Select(t="UI: Front Panel State >> Close", s=w603, f="") -> (s? t:f=w600:string)
        n223 = call <vilib>:"Add State(s) to Queue__jki_lib_state_machine.vi"("State(s) in (\"\")"=w600, "State(s) at Back (\"\")"="Data: Cleanup\nExit") -> ("States Out"=w598:string)  [unwired: 13 in]
        n224 = call <vilib>:"Add State(s) to Queue__jki_lib_state_machine.vi"("State(s) in Front (\"\")"=w598, "State(s) in (\"\")"=w607) -> ("States Out"=w606:string)  [unwired: 13 in]
      }
      frame "---------- Action ----------" {
        # "Template Separator\n(You can make a copy of, or modify, this frame)"
        n225 = call <vilib>:"Add State(s) to Queue__jki_lib_state_machine.vi"("State(s) in (\"\")"=w611) -> ("States Out"=w610:string)  [unwired: 14 in]
      }
      frame "Action: Find Callers" {
        # "#ToDo startup synchronization"
        # "This is used, because if Find Callers doesn't open it's FP before we finish running this VI, it will be garbage collected and never open. We should really be doing some startup synchronization."
        # "Template Separator\n(You can make a copy of, or modify, this frame)"
        n226 = Unbundle By Name(w622) -> ("JKI SM out"=w615:refnum<class "JKI SM.lvclass">, "States"=w621:string[])
        n227 = Scan From String(input string=w625, error in=w614, default 1=0 ("default value 1")) -> (output 1=w623:i32)  [unwired: 2 in, 3 out]
        n228 = Index Array(array=w621, index=w623) -> (element=w613:string)
        n229 = call <vilib>:"Parse State Queue__jki_lib_state_machine.vi"("State Queue"=w613) -> ("Current State"=w612:string)  [unwired: 12 in, 2 out]
        n230 = call "Find All Callers of State.vi"("error in (no error)"=w614, "State Name"=w612, "JKI SM in"=w615) -> ("error out"=w619:errorcluster, "Callers"=w620:T8, "JKI SM out"=w618:refnum<class "JKI SM.lvclass">)  [unwired: 6 in]
        n231 = call "Open Search Results Dialog.vi"("VI Refnum"=w616, "error in (no error)"=w619, "Callers"=w620, "State"=w612, "JKI SM in"=w618) -> ("error out"=w617:errorcluster)  [unwired: 6 in]
        n232 = call <vilib>:"Add State(s) to Queue__jki_lib_state_machine.vi"("State(s) in (\"\")"=w627) -> ("States Out"=w626:string)  [unwired: 14 in]
      }
    }
  }
  "error out" <- w3
